vi "LoadController.vi"(8 "error in (no error)":errorcluster, 10 "Actor In":refnum<class "Actor.lvclass">, 11 "DemoCamera in":refnum<class "DemoCamera.lvclass">) -> (0 "error out":errorcluster, 3 "DemoCamera out":refnum<class "DemoCamera.lvclass">)   [LabVIEW 2020, in "DemoCamera.lvlib" / "DemoCamera.lvclass"]
uses:
  DemoCamera.lvclass
  <vilib>/ActorFramework/Actor/Actor.lvclass
  ViewController/Prime95BCameraController/Prime95BCameraController.lvclass
  C:/Program Files/National Instruments/LabVIEW 2020/vi.lib/ActorFramework/Actor/Actor.lvclass
  Hardware Abstraction Layer/Component/Camera/Camera/Camera.lvclass
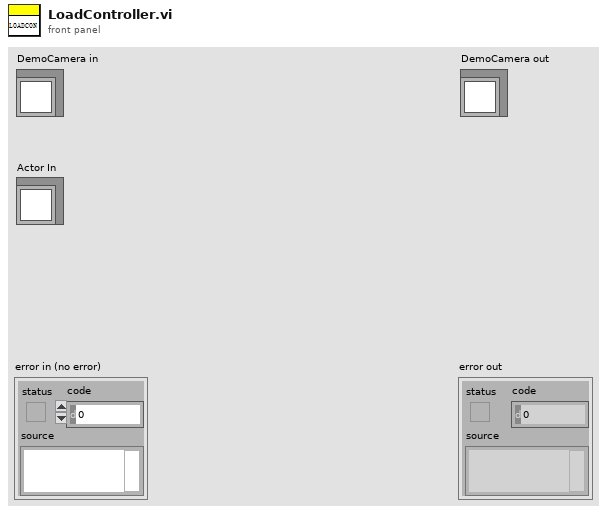
[diagram p1: front panel]
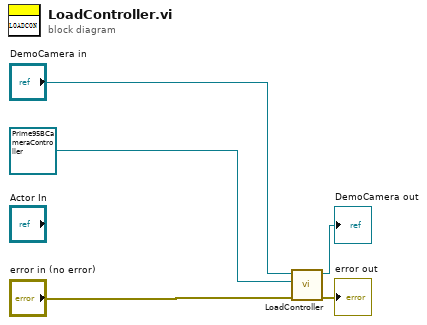
[diagram p0: block diagram]
diagram:
  n1 = call-parent "LoadController.vi"("error in (no error)"="error in (no error)", "Actor In"=refnum<class "Prime95BCameraController.lvclass"> refnum ("Prime95BCameraController.lvlib:Prime95BCameraController.lvclass"), "Device in"="DemoCamera in") -> ("error out"=→"error out":errorcluster, "Device out"=→"DemoCamera out":refnum<class "DemoCamera.lvclass">)  [unwired: 7 in]
